vi "RMS Simulation Test.vi"() -> ()   [LabVIEW 2014]
uses:
  <vilib>/Platform/TimedLoop/XDataNode/timing_clust.ctl
  <vilib>/Platform/TimedLoop/XDataNode/nitl_modes.ctl
  <vilib>/Platform/TimedLoop/XDataNode/wakeup.ctl
  <vilib>/rvi/FXPMathLib/basic elements/FxpIntAccumulator/subVIs/nifxpmath_IntAccumulator_SimConfig.ctl
  <vilib>/rvi/FXPMathLib/FxpSqrt/subVIs/nifxpmath_Sqrt_SimConfig.ctl
  <vilib>/fxp/LVFixedPointOverflowPolicyTypeDef.ctl
  <vilib>/rvi/Emulation/niFpgaSctlEmulationGetInTimedLoop.vi
  <vilib>/rvi/Emulation/niFpgaEmulationReportErrorSimple.vi
  <vilib>/rvi/Emulation/niFpgaGetClockAttributes.vi
  <vilib>/rvi/Emulation/niFpgaCriticalErrorInLSC.vi
  <vilib>/rvi/Memory/Memory_Emulation/nirvimemoryFastEmulation.vi
  <vilib>/rvi/Memory/Memory_Emulation/nirvimemoryEmulation.vi
  <vilib>/rvi/Emulation/niFpgaEmulationIsFPGAContextNoSignature.vi
  <vilib>/rvi/DataTransferAndStorage/Container/Common/niFpgaContainerGetUniqueNameForEmu.vi
  <vilib>/rvi/Emulation/niFpgaProcessEmulError.vi
  <vilib>/rvi/errors/nirviReportUnexpectedCaseInternalError (U32).vi
  <vilib>/rvi/errors/niFpgaSetErrorForExecOnDevCompSimple.vi
  <vilib>/rvi/eio/common/nirviEmuReportErrorAndStop.vi
  <vilib>/rvi/FIFO/Fifo_Resource/nirvififoEmulationSetSize.vi
  <vilib>/rvi/FIFO/Fifo_Resource/nirviFifoEmulationQueueMgr.vi
  <instcachedir>/0/nirviFifoEmulationQueueMgr_E5CAEC123FF24DC58D834DCA3CDAA9B5.lvgen/nirviFifoEmulationQueueMgr_E5CAEC123FF24DC58D834DCA3CDAA9B5_010.vi
  <vilib>/rvi/FIFO/Fifo_Resource/nirvififoEmulationDetermineInputValidOut.vi
  <vilib>/rvi/FIFO/Fifo_Resource/nirvififoEmulationCreateLock.vi
  <vilib>/rvi/FIFO/Fifo_Resource/nirvififoEmulationObtainLock.vi
  <vilib>/rvi/FIFO/Fifo_Resource/nirvififoEmulationReleaseLock.vi
  <vilib>/rvi/occurrence/nirviWaitOnOccurrenceBase.vi
  <vilib>/rvi/errors/nirviReportUnexpectedCaseInternalError.vi
  <vilib>/rvi/Analysis/common/codeGenErrors/XNode/niFpgaXNodeCodeGenErrorHandle.vi
  <vilib>/rvi/FXPMathLib/basic elements/FxpIntAccumulator/simVIs/DllFxpIntAccumulator_sub.vi
  <vilib>/rvi/FXPMathLib/FxpSqrt/simVIs/DllSqrtTemp_sub.vi
  <vilib>/Platform/TimedLoop/XDataNode/XDataNode.xnode
  <vilib>/rvi/DataTransferAndStorage/Container/XNode/niFpgaContainer.xnode
  <vilib>/rvi/FIFO/Fifo_Resource/nirvififoEmulationWrite.vi
  <vilib>/rvi/FIFO/Fifo_Resource/nirvififoEmulationRead.vi
  <vilib>/rvi/Analysis/measure/dc-rms/XNode/niFpgaDC-RMS.xnode
  <vilib>/rvi/FXPMathLib/FxpMul/XNode/nifxpmath_Multiplier.xnode
  <vilib>/rvi/FXPMathLib/basic elements/FxpIntAccumulator/XNode/nifxpmath_IntAccumulator.xnode
  <vilib>/rvi/FXPMathLib/FxpSqrt/XNode/nifxpmath_Sqrt.xnode
  <vilib>/Platform/TimedLoop/XDataNode/XDNodeRunTimeDep.lvlib
  <vilib>/rvi/FXPMathLib/sim/FxpSim.dll
panel:
  out "DC":fxp<+/-,12,12>
  out "RMS":fxp<+,12,12>
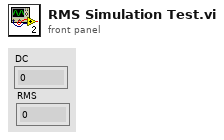
[diagram p1: front panel]
types:
  T1 = typedef "XDNodeRunTimeDep.lvlib/timing_clust.ctl" = cluster{"Expected End [f-1]":u64, "Actual End [f-1]":u64, "Finished Late? [f-1]":bool, "Expected End [i-1]":u64, "Actual End [i-1]":u64, "Finished Late? [i-1]":bool, "Expected Start [i]":u64, "Actual Start [i]":u64, "Expected Start [f]":u64, "Actual Start [f]":u64, "Source Name":string, "Structure Name":string, "Period":i64, "Deadline":i64, "Offset":i64, "Start":i64, "Priority":i32, "Timeout":i32, "Mode":T2, "Wakeup Reason":T3, "Error":errorcluster, "Source Type":string, "Secondary Source Type":string, "Global End Time":u64, "Global Start Time":u64, "Frame Duration":u64, "Iteration Duration":u64, "Assigned CPU":i32, "I/O Scan Engine Mode":u32}
  T2 = typedef "XDNodeRunTimeDep.lvlib/nitl_modes.ctl" = enum32{"No Change", "Process missed periods, maintain original phase", "Discard missed periods, maintain original phase", "Process missed periods, ignore original phase", "Discard missed periods, ignore original phase"}
  T3 = typedef "XDNodeRunTimeDep.lvlib/wakeup.ctl" = enum32{"Normal", "Aborted", "Asynchronous wakeup", "Timing source error", "Timed loop error", "Timeout"}
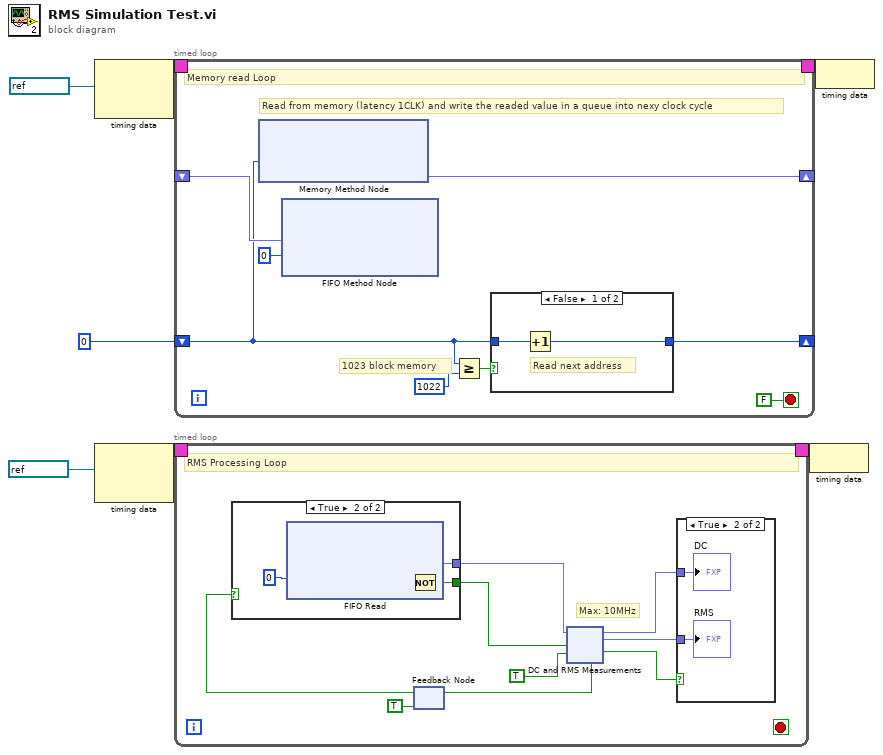
[diagram p0: block diagram]
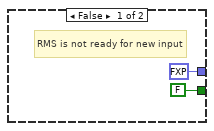
[diagram p3: hidden frame]
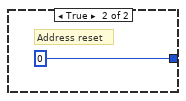
[diagram p4: hidden frame]
diagram:
  n1 = node-c288(refnum<k21> "10MHz" ("Source Name")) -> (w7:T1)  [unwired: 1 in]
  n2 = node-c288(refnum<k21> "10MHz" ("Source Name")) -> (w5:T1)  [unwired: 1 in]
  n3 = timed-loop {
    timing: w7 -> [_]
    timing-out: [_] -> w6
    shift-right: [w15] -> _
    shift-left: _ -> [w11]
    shift-right: [w12] -> _
    shift-left: u32 0 -> [w8]
    stop <- FALSE stop-if-true
    # "1023 block memory"
    # "Read from memory (latency 1CLK) and write the readed value in a queue into nexy clock cycle"
    # "Memory read Loop"
    n4 = xnode ("Memory Method Node")("Address"=w8) -> ("Data"=w15:fxp<+/-,12,12>)  [unwired: 1 in, 1 out]
    n5 = xnode ("FIFO Method Node")("Element"=w11, "Timeout"=0) -> ()  [unwired: 1 in, 2 out]
    n6 = Greater Or Equal?(x=w8, y=u32 1022) -> (x >= y?=w13:bool)
    n7 = case shown="False" w13 {
      tunnel: w8 -> [w17 _]
      tunnel: [w16 u32 0] -> w12
      frame False {
        # "Read next address"
        n8 = Increment(x=w17) -> (x+1=w16:u32)
      }
      frame True {
        # "Address reset"
      }
    }
  }
  n9 = timed-loop {
    timing: w5 -> [_]
    timing-out: [_] -> w4
    stop <- _ stop-if-true
    # "Max: 10MHz"
    # "RMS Processing Loop"
    n10 = feedback #1(TRUE ("ready for input")) -> (w29:bool)
    n11 = case shown="True" w29 {
      tunnel: [FALSE w188] -> w25
      tunnel: [fxp<+/-,12,12> 0.0 ("Element") w185] -> w21
      frame False {
        # "RMS is not ready for new input"
      }
      frame True {
        n12 = xnode ("FIFO Read")("Timeout"=0) -> ("Element"=w185:fxp<+/-,12,12>, "Timed Out?"=w187:bool)  [unwired: 1 in, 1 out]
        n13 = Not(x=w187) -> (.not. x?=w188:bool)
      }
    }
    n14 = xnode "DC and RMS Measurements"("input data"=w21, "input valid"=w25, "ready for output"=TRUE) -> ("DC"=w23:fxp<+/-,12,12>, "RMS"=w22:fxp<+,12,12>, "output valid"=w27:bool, "ready for input"=w26:bool)  [unwired: 1 in]
    n15 = feedback-in #1(w26) -> ()
    n16 = case shown="True" w27 {
      tunnel: w23 -> [_ w182]
      tunnel: w22 -> [_ w181]
      frame False {
      }
      frame True {
        "DC" <- w182
        "RMS" <- w181
      }
    }
  }
  n17 = node-c288(w4) -> ()
  n18 = node-c288(w6) -> ()
